vi "Set Power.vi"(8 "error in (no error)":errorcluster, 9 "Channel":i32, 10 "Power (dBm)":dbl, 11 "Instrument.VSource in":refnum<class "VNA.lvclass">) -> (0 "error out":errorcluster, 3 "Instrument.VSource out":refnum<class "VNA.lvclass">)   [LabVIEW 2019, in "VNA.lvclass"]
uses:
  VNA.lvclass
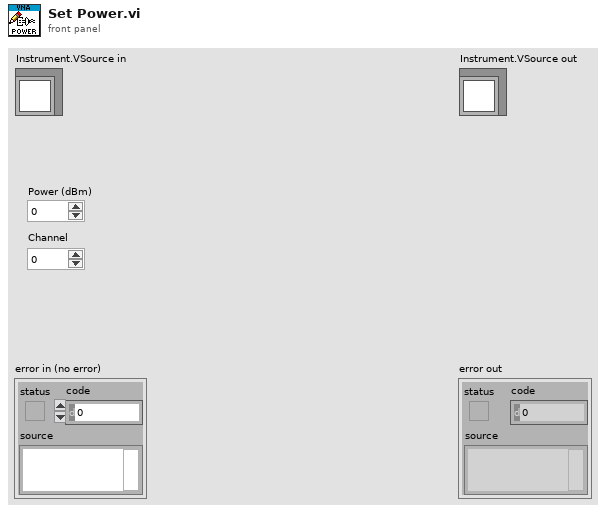
[diagram p1: front panel]
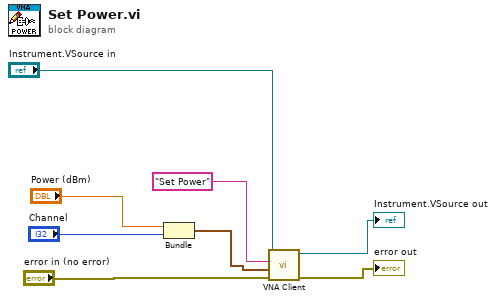
[diagram p0: block diagram]
diagram:
  n1 = Bundle("Power (dBm)"="Power (dBm)", "Channel"="Channel") -> (w2:cluster{"Power (dBm)":dbl, "Channel":i32})  [unwired: 1 in]
  n2 = call "VNA Client.vi"("error in (no error)"="error in (no error)", "Data"=w2, "Command"="Set Power", "VNA in"="Instrument.VSource in") -> ("error out"=→"error out":errorcluster, "VNA out"=→"Instrument.VSource out":refnum<class "VNA.lvclass">)  [unwired: 6 in]
